vi "Receiving_Process (SubVI).vi"(10 "value in":string[](array[string]), 11 "Digital in":refnum<vi>) -> (1 "Array":string[](array[string]), 2 "Array 2":string[](array[string]), 3 "Boolean":bool)   [LabVIEW 2019]
uses:
  <vilib>/numeric/Random Number (Range) DBL.vi
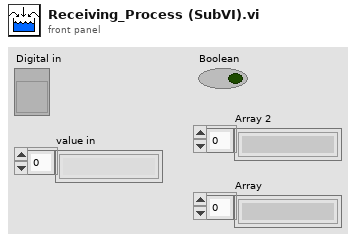
[diagram p1: front panel]
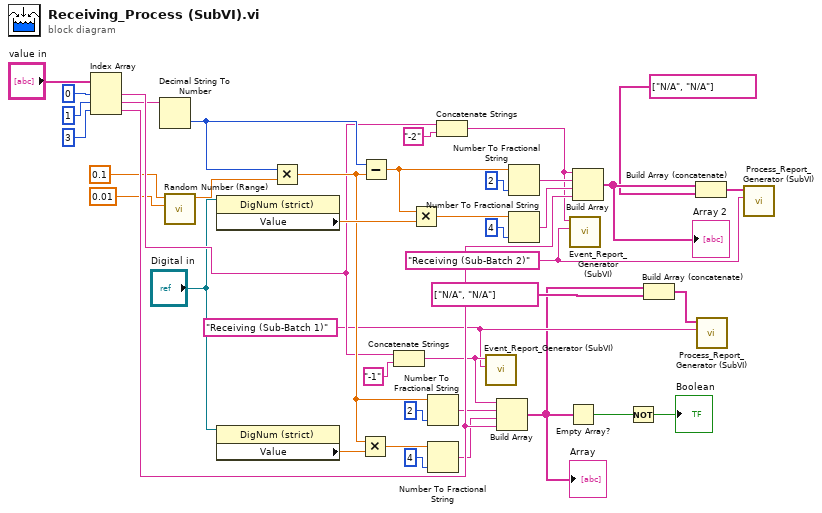
[diagram p0: block diagram]
diagram:
  w7 = "Receiving (Sub-Batch 1)" ("Process Name")
  w8 = "Receiving (Sub-Batch 2)" ("Process Name")
  n1 = Index Array(array="value in", index #1=0 ("index"), index #2=1 ("index"), index #3=3 ("index")) -> (element #1=w29:string, element #2=w27:string, element #3=w37:string)
  n2 = Decimal String To Number(string=w27) -> (number=w30:i32)  [unwired: 2 in, 1 out]
  n3 = call-poly <vilib>:"Random Number (Range).vi"("lower bound (0)"=0.01, "upper bound (100)"=0.1) -> ("number"=w19:dbl)  [unwired: 9 in]
  n4 = property class="DigNum (strict)"(reference="Digital in") -> ("Value"=w39:dbl)  [unwired: 1 in, 2 out]
  n5 = property class="DigNum (strict)"(reference="Digital in") -> ("Value"=w20:dbl)  [unwired: 1 in, 2 out]
  n6 = Multiply(x=w30, y=w19) -> (x*y=w38:dbl)
  n7 = Multiply(x=w38, y=w20) -> (x*y=w21:dbl)
  n8 = Subtract(x=w30, y=w38) -> (x-y=w40:dbl)
  n9 = Concatenate Strings(w29, "-1" ("string")) -> (w9:string)
  n10 = Multiply(x=w40, y=w39) -> (x*y=w34:dbl)
  n11 = Number To Fractional String(number=w38, precision (6)=i16 2) -> (F-format string=w22:string)  [unwired: 2 in]
  n12 = Number To Fractional String(number=w21, precision (6)=i16 4) -> (F-format string=w23:string)  [unwired: 2 in]
  n13 = Concatenate Strings(w29, "-2" ("string")) -> (w10:string)
  n14 = call "Event_Report_Generator (SubVI).vi"("Process Name"=w7, "Booking ID"=w9) -> ()  [unwired: 10 in]
  n15 = Build Array(w9, w22, w23, w37) -> (w2:string[])
  "Array" <- w2
  n16 = Number To Fractional String(number=w40, precision (6)=i16 2) -> (F-format string=w32:string)  [unwired: 2 in]
  n17 = Number To Fractional String(number=w34, precision (6)=i16 4) -> (F-format string=w35:string)  [unwired: 2 in]
  n18 = Empty Array?(array=w2) -> (empty?=w26:bool)
  n19 = call "Event_Report_Generator (SubVI).vi"("Process Name"=w8, "Booking ID"=w10) -> ()  [unwired: 10 in]
  n20 = Build Array(w10, w32, w35, w37) -> (w6:string[])
  "Array 2" <- w6
  n21 = Not(x=w26) -> (.not. x?=→"Boolean":bool)
  n22 = Build Array (concatenate)(w2, string[] ["N/A", "N/A"] ("array")) -> (w1:string[])
  n23 = Build Array (concatenate)(w6, string[] ["N/A", "N/A"] ("array")) -> (w4:string[])
  n24 = call "Process_Report_Generator (SubVI).vi"("Process Name"=w7, "Process Information"=w1) -> ()  [unwired: 10 in]
  n25 = call "Process_Report_Generator (SubVI).vi"("Process Name"=w8, "Process Information"=w4) -> ()  [unwired: 10 in]
